vi "USB2CAN_UDSTest .vi"() -> ()   [LabVIEW 2010]
panel:
  in  "Baudrate":u32(ring)=500000 items=["1000 Kbps"=1000000, "500 Kbps"=500000, "250 Kbps"=250000, "200 Kbps"=200000, "125 Kbps"=125000, "100 Kbps"=100000, ""=0]
  in  "pUDSAddr":T1={"ReqID"=1793, "ResID"=601, "Flag"=0, "AddrFormats"=0, "AddrExt"=0, "MaxDLC"=8} {"ReqID" format="%x"}
  in  "pResData":u8[](array[numeric])=array[4097 elements]
  out "pResData out":u8[](array[numeric])
  in  "pReqData":u8[](array[numeric])=array[4097 elements] format="%x"
  out "pReqData out":u8[](array[numeric])
  out "pUDSAddr out":T2
  in  "stop":bool
  in  "pCanConfig":T3={"CAN_BRP"=4, "CAN_SJW"=1, "CAN_BS1"=15, "CAN_BS2"=5, "CAN_Mode"=128, "CAN_ABOM"=1, "CAN_NART"=0, "CAN_RFLM"=0, "CAN_TXFP"=1} {"CAN_Mode" format="%x"}
  in  "Send Channel":u8(ring) items=["CAN1", "CAN2"]
  in  "Device Index":i32(ring) items=["0", "1", "2", "3", "4", "5"]
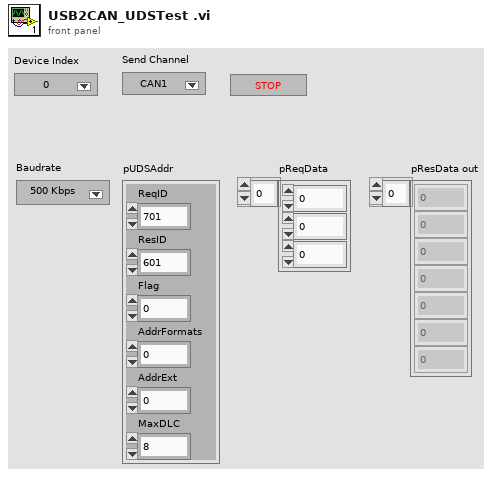
[diagram p1: front panel]
types:
  T1 = cluster{"ReqID":u32, "ResID":u32, "Flag":u8, "AddrFormats":u8, "AddrExt":u8, "MaxDLC":u8}
  T2 = cluster{"ReqID":u32, "ResID":u32, "ExternFlag":u8, "AddrFormats":u8, "AddrExt":u8, "__Res":u8}
  T3 = cluster{"CAN_BRP":u32, "CAN_SJW":u8, "CAN_BS1":u8, "CAN_BS2":u8, "CAN_Mode":u8, "CAN_ABOM":u8, "CAN_NART":u8, "CAN_RFLM":u8, "CAN_TXFP":u8}
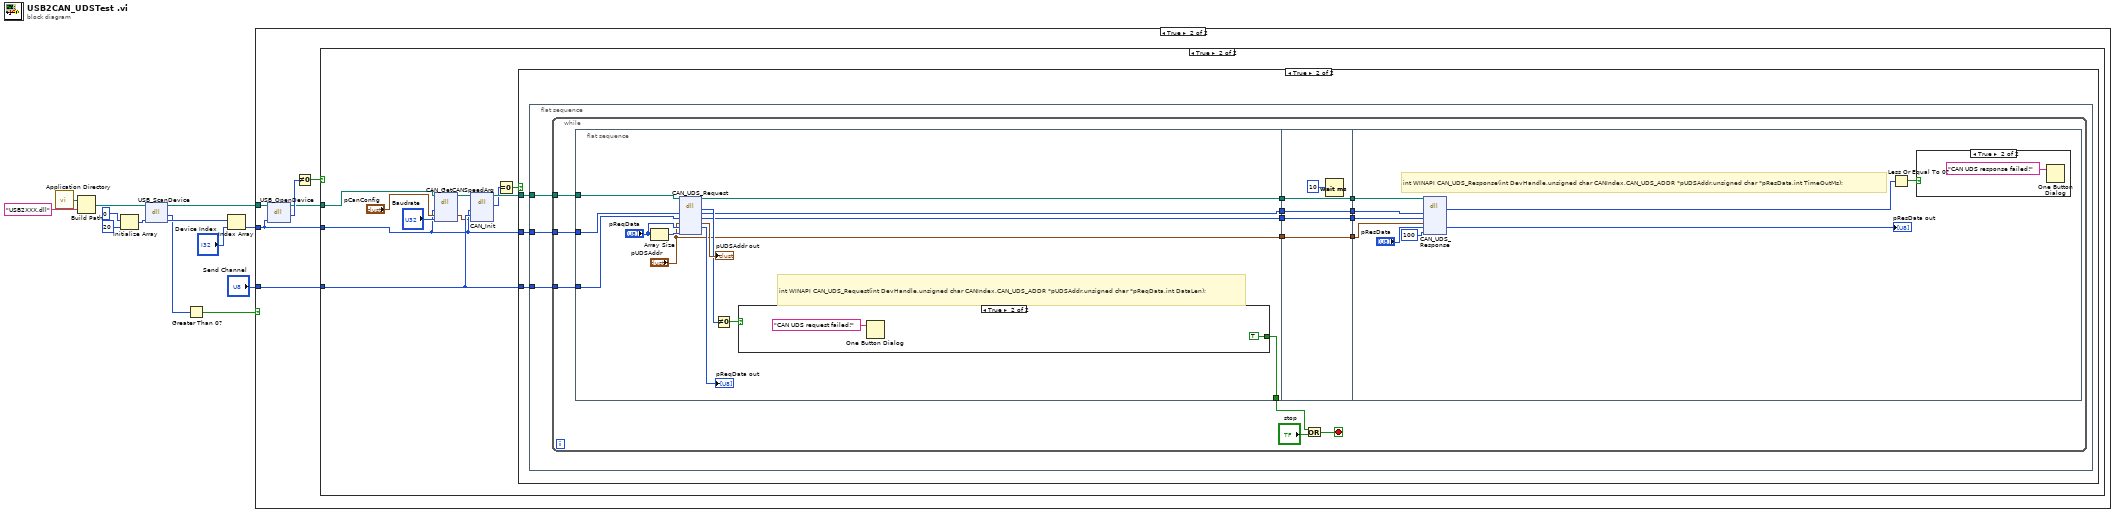
[diagram p0: block diagram]
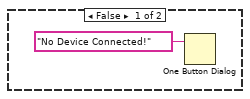
[diagram p2: hidden frame]
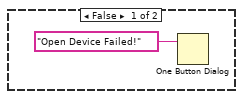
[diagram p3: hidden frame]
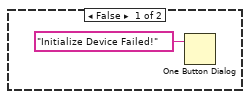
[diagram p4: hidden frame]
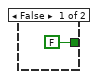
[diagram p5: hidden frame]
diagram:
  n1 = call <vilib>:"Application Directory.vi"() -> ("Application Directory"=w2:path)
  n2 = Build Path(base path=w2, name or relative path="USB2XXX.dll") -> (appended path=w1:path)
  n3 = Initialize Array(0, 20 ("dimension size")) -> (w13:i32[])
  n4 = dll-call lib="E:/OtherWork/STM32/USB2XXX_Example/sdk/api/Labview/USB2XXX.dll" fn="USB_ScanDevice"(path in=w1, "pDevNum"=w13) -> (path out=w4:path, "return type"=w9:i32, "pDevNum"=w10:i32[])  [unwired: 2 in, 1 out]
  n5 = Greater Than 0?(x=w9) -> (x > 0?=w8:bool)
  n6 = Index Array(array=w10, index="Device Index") -> (element=w6:i32)
  n7 = case shown="True" w8 {
    tunnel: w6 -> [_ w17]
    tunnel: w4 -> [_ w18]
    tunnel: "Send Channel" -> [_ w16]
    frame False {
      n8 = One Button Dialog(message="No Device Connected!") -> ()  [unwired: 1 in, 1 out]
    }
    frame True {
      n9 = dll-call lib="E:/OtherWork/STM32/USB2XXX_Example/sdk/api/Labview/USB2XXX.*" fn="USB_OpenDevice"(path in=w18, "DevHandle"=w17) -> (path out=w15:path, "return type"=w20:u8)  [unwired: 3 in, 1 out]
      n10 = Not Equal To 0?(x=w20) -> (x != 0?=w19:bool)
      n11 = case shown="True" w19 {
        tunnel: w15 -> [_ w27]
        tunnel: w17 -> [_ w23]
        tunnel: w16 -> [_ w30]
        frame False {
          n12 = One Button Dialog(message="Open Device Failed!") -> ()  [unwired: 1 in, 1 out]
        }
        frame True {
          n13 = dll-call lib="E:/Projects/USB2XXX_Example/sdk/api/Labview/usb2can/USB2XXX.*" fn="CAN_GetCANSpeedArg"(path in=w27, "DevHandle"=w23, "pCanConfig"="pCanConfig", "SpeedBps"="Baudrate") -> (path out=w26:path, "pCanConfig"=w22:T3)  [unwired: 5 in, 1 out]
          n14 = dll-call lib="E:/OtherWork/STM32/USB2XXX_Example/sdk/api/Labview/USB2XXX.*" fn="CAN_Init"(path in=w26, "DevHandle"=w23, "CANIndex"=w30, "pCanConfig"=w22) -> (path out=w31:path, "return type"=w29:i32)  [unwired: 5 in, 1 out]
          n15 = Equal To 0?(x=w29) -> (x = 0?=w28:bool)
          n16 = case shown="True" w28 {
            tunnel: w31 -> [_ w33]
            tunnel: w23 -> [_ w34]
            tunnel: w30 -> [_ w35]
            frame False {
              n17 = One Button Dialog(message="Initialize Device Failed!") -> ()  [unwired: 1 in, 1 out]
            }
            frame True {
              n18 = flat-sequence {
                tunnel: w33 -> [w38]
                tunnel: w35 -> [w37]
                tunnel: w34 -> [w36]
                frame #0 {
                  n19 = while {
                    tunnel: w38 -> [w52]
                    tunnel: w37 -> [w51]
                    tunnel: w36 -> [w50]
                    stop <- w40 stop-if-true
                    n20 = flat-sequence {
                      tunnel: w52 -> [w58]
                      tunnel: w51 -> [w63]
                      tunnel: w50 -> [w64]
                      tunnel: [w57] -> w48
                      tunnel: [w56] -> w46
                      tunnel: [w55] -> w44
                      tunnel: ["pUDSAddr"] -> w42
                      tunnel: [w53] -> w39
                      tunnel: [w73] -> w49
                      tunnel: w48 -> [w73]
                      tunnel: [w72] -> w47
                      tunnel: w46 -> [w72]
                      tunnel: [w71] -> w45
                      tunnel: w44 -> [w71]
                      tunnel: [w70] -> w43
                      tunnel: w42 -> [w70]
                      tunnel: w49 -> [w81]
                      tunnel: w47 -> [w80]
                      tunnel: w45 -> [w79]
                      tunnel: w43 -> [w78]
                      frame #0 {
                        # "int WINAPI CAN_UDS_Request(int DevHandle,unsigned char CANIndex,CAN_UDS_ADDR *pUDSAddr,unsigned char *pReqData,int DataLen);"
                        n21 = Array Size(array="pReqData") -> (size(s)=w62:i32)
                        n22 = dll-call lib="E:/OtherWork/STM32/USB2XXX/trunk/USB2XXX/USB2XXX/vs2010/Release/USB2XXX.*" fn="CAN_UDS_Request"(path in=w58, "DevHandle"=w64, "CANIndex"=w63, "pUDSAddr"="pUDSAddr", "pReqData"="pReqData", "DataLen"=w62) -> (path out=w57:path, "return type"=w60:i32, "DevHandle"=w56:i32, "CANIndex"=w55:u8, "pUDSAddr"=→"pUDSAddr out":T1, "pReqData"=→"pReqData out":u8[])  [unwired: 3 in, 1 out]
                        n23 = Not Equal To 0?(x=w60) -> (x != 0?=w59:bool)
                        n24 = case shown="True" w59 {
                          tunnel: [FALSE TRUE] -> w53
                          frame False {
                          }
                          frame True {
                            n25 = One Button Dialog(message="CAN UDS request failed!") -> ()  [unwired: 1 in, 1 out]
                          }
                        }
                      }
                      frame #1 {
                        n26 = Wait (ms)(milliseconds to wait=u32 10 ("等待时间（毫秒）")) -> ()  [unwired: 1 out]
                      }
                      frame #2 {
                        # "int WINAPI CAN_UDS_Response(int DevHandle,unsigned char CANIndex,CAN_UDS_ADDR *pUDSAddr,unsigned char *pResData,int TimeOutMs);"
                        n27 = dll-call lib="E:/OtherWork/STM32/USB2XXX/trunk/USB2XXX/USB2XXX/vs2010/Release/USB2XXX.*" fn="CAN_UDS_Response"(path in=w81, "DevHandle"=w80, "CANIndex"=w79, "pUDSAddr"=w78, "pResData"="pResData", "TimeOutMs"=100) -> ("return type"=w76:i32, "pResData"=→"pResData out":u8[])  [unwired: 6 in, 2 out]
                        n28 = Less Or Equal To 0?(x=w76) -> (x <= 0?=w75:bool)
                        n29 = case shown="True" w75 {
                          frame False {
                          }
                          frame True {
                            n30 = One Button Dialog(message="CAN UDS response failed!") -> ()  [unwired: 1 in, 1 out]
                          }
                        }
                      }
                    }
                    n31 = Or(x=w39, y="stop") -> (x .or. y?=w40:bool)
                  }
                }
              }
            }
          }
        }
      }
    }
  }
